vi "最大权值.vi"(0 "白子棋盘权值":sgl[][](array[numeric]), 5 "黑子棋盘权值":sgl[][](array[numeric])) -> (4 "权值最大的前三个位置":dbl[][](array[numeric]), 8 "白子权值勤大于黑子？":bool, 10 "白子最大权值":sgl, 15 "黑子最大权值":sgl)   [LabVIEW 2018]
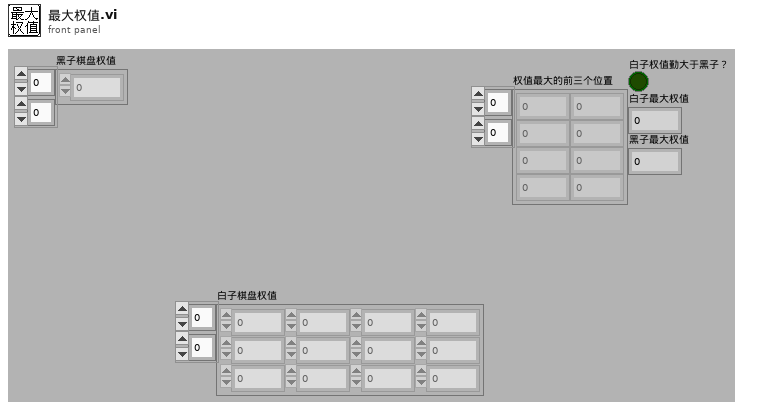
[diagram p1: front panel]
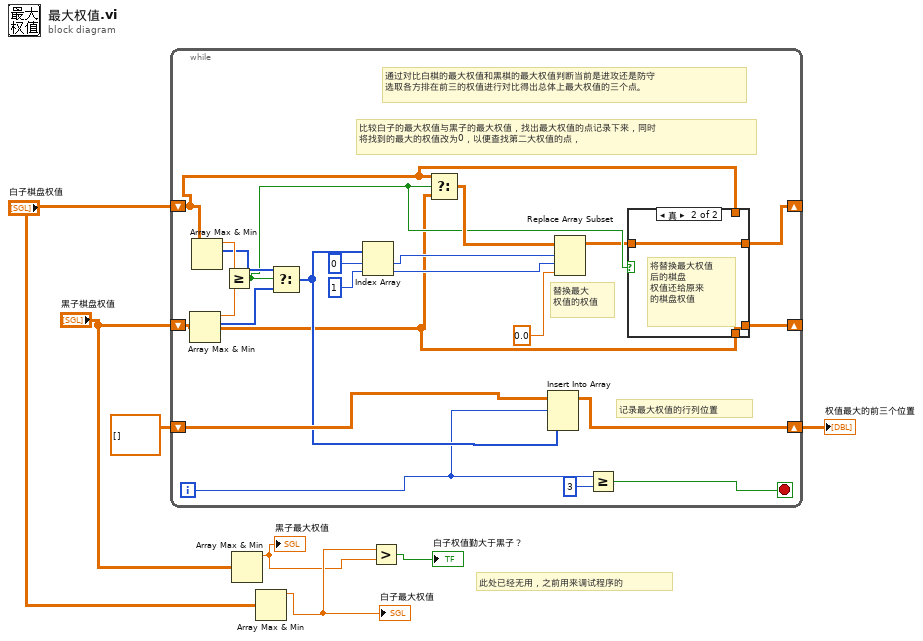
[diagram p0: block diagram]
diagram:
  # "此处已经无用，之前用来调试程序的"
  n1 = while {
    shift-right: [w12] -> _
    shift-left: "白子棋盘权值" -> [w10]
    shift-right: [w23] -> w6
    shift-left: dbl[][] [] ("array") -> [w22]
    shift-right: [w11] -> _
    shift-left: "黑子棋盘权值" -> [w9]
    i -> [w8]
    stop <- w25 stop-if-true
    # "记录最大权值的行列位置"
    # "替换最大\n权值的权值"
    # "比较白子的最大权值与黑子的最大权值，找出最大权值的点记录下来，同时\n将找到的最大的权值改为0，以便查找第二大权值的点，"
    # "通过对比白棋的最大权值和黑棋的最大权值判断当前是进攻还是防守\n选取各方排在前三的权值进行对比得出总体上最大权值的三个点。"
    n2 = Array Max & Min(array=w9) -> (max value=w19:sgl, max index (indices)=w17:i32[])  [unwired: 2 out]
    n3 = Array Max & Min(array=w10) -> (max value=w20:sgl, max index (indices)=w18:i32[])  [unwired: 2 out]
    n4 = Greater Or Equal?(x=w20, y=w19) -> (x >= y?=w14:bool)
    n5 = Select(t=w18, s=w14, f=w17) -> (s? t:f=w16:i32[])
    n6 = Index Array(array=w16, index #1=0 ("index"), index #2=1 ("index")) -> (element #1=w27:i32, element #2=w26:i32)
    n7 = Select(t=w10, s=w14, f=w9) -> (s? t:f=w15:sgl[][])
    n8 = Insert Into Array(array=w22, index (row)=w8, new element=w16) -> (w23:dbl[][])  [unwired: 1 in]
    n9 = Replace Array Subset(array=w15, new element=sgl 0.0 ("new element/subarray"), index (row)=w27, index (col)=w26) -> (w13:sgl[][])
    n10 = Greater Or Equal?(x=w8, y=3) -> (x >= y?=w25:bool)
    n11 = case shown="真" w14 {
      tunnel: w13 -> [w31 w33]
      tunnel: [w30 w33] -> w12
      tunnel: [w31 w32] -> w11
      tunnel: w10 -> [w30 _]
      tunnel: w9 -> [_ w32]
      frame False {
        # "将替换最大权值\n后的棋盘\n权值还给原来\n的棋盘权值"
      }
      frame True {
        # "将替换最大权值\n后的棋盘\n权值还给原来\n的棋盘权值"
      }
    }
  }
  "权值最大的前三个位置" <- w6
  n12 = Array Max & Min(array="黑子棋盘权值") -> (max value=w1:sgl)  [unwired: 3 out]
  "黑子最大权值" <- w1
  n13 = Array Max & Min(array="白子棋盘权值") -> (max value=w2:sgl)  [unwired: 3 out]
  "白子最大权值" <- w2
  n14 = Greater?(x=w2, y=w1) -> (0:→"白子权值勤大于黑子？":bool)
